vi "Get Size of Data from TD - Benchmark Array of Fixed-size Type (DBL) - Should Perform in O(1).vi"() -> ()   [LabVIEW 2017, in "Composition.Tests.lvlib"]
uses:
  Composition.Tests.lvlib
  <vilib>/addons/_JKI Toolkits/Caraya/classes/Assert/Assert Less_Variant.vi
  Composition/Composition.lvlib
  <vilib>/addons/_JKI Toolkits/Caraya/classes/Test/Test.lvclass
  <vilib>/addons/_JKI Toolkits/Caraya/classes/Assert/Assert.lvclass
panel:
  out "error out":errorcluster
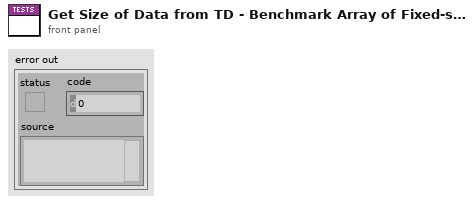
[diagram p1: front panel]
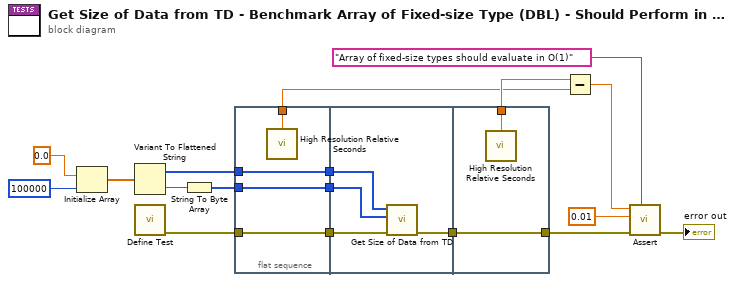
[diagram p0: block diagram]
diagram:
  n1 = Initialize Array(0.0 ("element"), 100000 ("dimension size")) -> (w16:dbl[])
  n2 = Variant To Flattened String(Variant=w16) -> (data string=w15:string, 1:w14:i16[])
  n3 = call <vilib>:"Define Test.vi"() -> ("error out"=w12:errorcluster)  [unwired: 11 in]
  n4 = String To Byte Array(string=w15) -> (unsigned byte array=w13:u8[])
  n5 = flat-sequence {
    tunnel: w12 -> [w20]
    tunnel: w13 -> [w21]
    tunnel: w14 -> [w22]
    tunnel: [w22] -> w11
    tunnel: [w21] -> w10
    tunnel: [w20] -> w9
    tunnel: [w19] -> w7
    tunnel: w11 -> [w26]
    tunnel: w10 -> [w25]
    tunnel: w9 -> [w24]
    tunnel: [w23] -> w6
    tunnel: [w28] -> w8
    tunnel: [w27] -> w5
    tunnel: w6 -> [w27]
    frame #0 {
      n6 = call <vilib>:"High Resolution Relative Seconds.vi"() -> ("relative seconds"=w19:dbl)
    }
    frame #1 {
      n7 = call "Get Size of Data from TD.vi"("error in (no error)"=w24, "Data String"=w25, "Type Descriptor"=w26) -> ("error out"=w23:errorcluster)  [unwired: 7 in, 1 out]
    }
    frame #2 {
      n8 = call <vilib>:"High Resolution Relative Seconds.vi"() -> ("relative seconds"=w28:dbl)
    }
  }
  n9 = Subtract(x=w8, y=w7) -> (x-y=w4:dbl)
  n10 = call-poly <vilib>:"Assert.vi"("Label"="Array of fixed-size types should evaluate in O(1)", "error in (no error)"=w5, "Y"=0.01 ("x-y"), "X"=w4) -> ("error out"=→"error out":errorcluster)  [unwired: 7 in]
